vi "EV Rotator Shutdown Editor.vi"(6 "Channel":i32=1, 8 "Calibration in":string, 9 "Hardware in":string, 10 "Setup in":string, 11 "Editor seq info":T1 {"Steps config"."Loop Info"."unit scale" items=["Log", "Lin"]; "Steps config"."Loop Info"."unit dB ref" format="%#_6p"}) -> (1 "Step name out":string="Calibration Default", 2 "Setup out":string, 3 "Sequence channels & curves out":string[](array[string]))   [LabVIEW 2018]
uses:
  custom and Sc run Seq Sub VIs (x64).llb/editor seq info.ctl
  custom and Sc run Seq Sub VIs (x64).llb/Steps config.ctl
  C:/SoundCheck 19/System/Custom VIs/EV.Rotator.RotatorControl.dll
  EV.Rotator.RotatorControl.dll
panel:
  out "Rotator Control.dll version":string
  in  "Save as":bool
  in  "save":bool
  in  "revert":bool
  in  "continue loop?":bool
  in  "cancel":bool
  in  "load":bool
  # "This VI runs the following shutdown routine:\n  - disables absolute movement mode\n  - disables drives\n  - enables Ab mode\n  - disables Ab mode"
  # "Reminder:  You must edit this custom step from\nwithin a sequence for it to remember your settings."
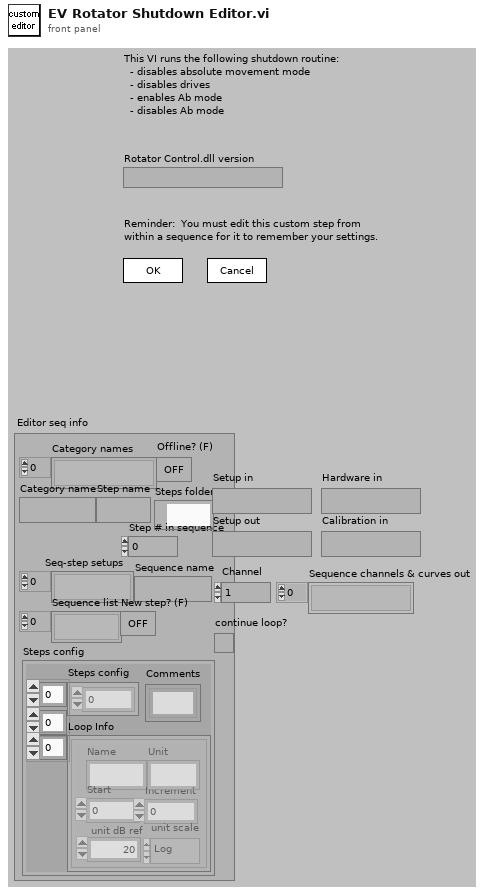
[diagram p1: front panel]
types:
  T1 = typedef "editor seq info.ctl" = cluster{"Category names":string[], "Category name":string, "Step name":string, "Step # in sequence":i32, "Seq-step setups":string[], "Sequence name":string, "Sequence list":string[], "New step? (F)":bool, "Steps config":T2, "Offline? (F)":bool, "Steps folder":path}
  T2 = typedef "Steps config.ctl" = cluster{"Steps config":i32[][], "Loop Info":cluster{"Name":string, "Start":dbl, "Increment":dbl, "Unit":string, "unit dB ref":dbl, "unit scale":u16}[], "Comments":string[]}
  T3 = cluster{"load":bool, "revert":bool, bool, "cancel":bool, "Save as":bool, bool, bool}
  T4 = cluster{"load":bool, "revert":bool, "save":bool, "cancel":bool, "Save as":bool, "close panel":bool, "apply":bool}
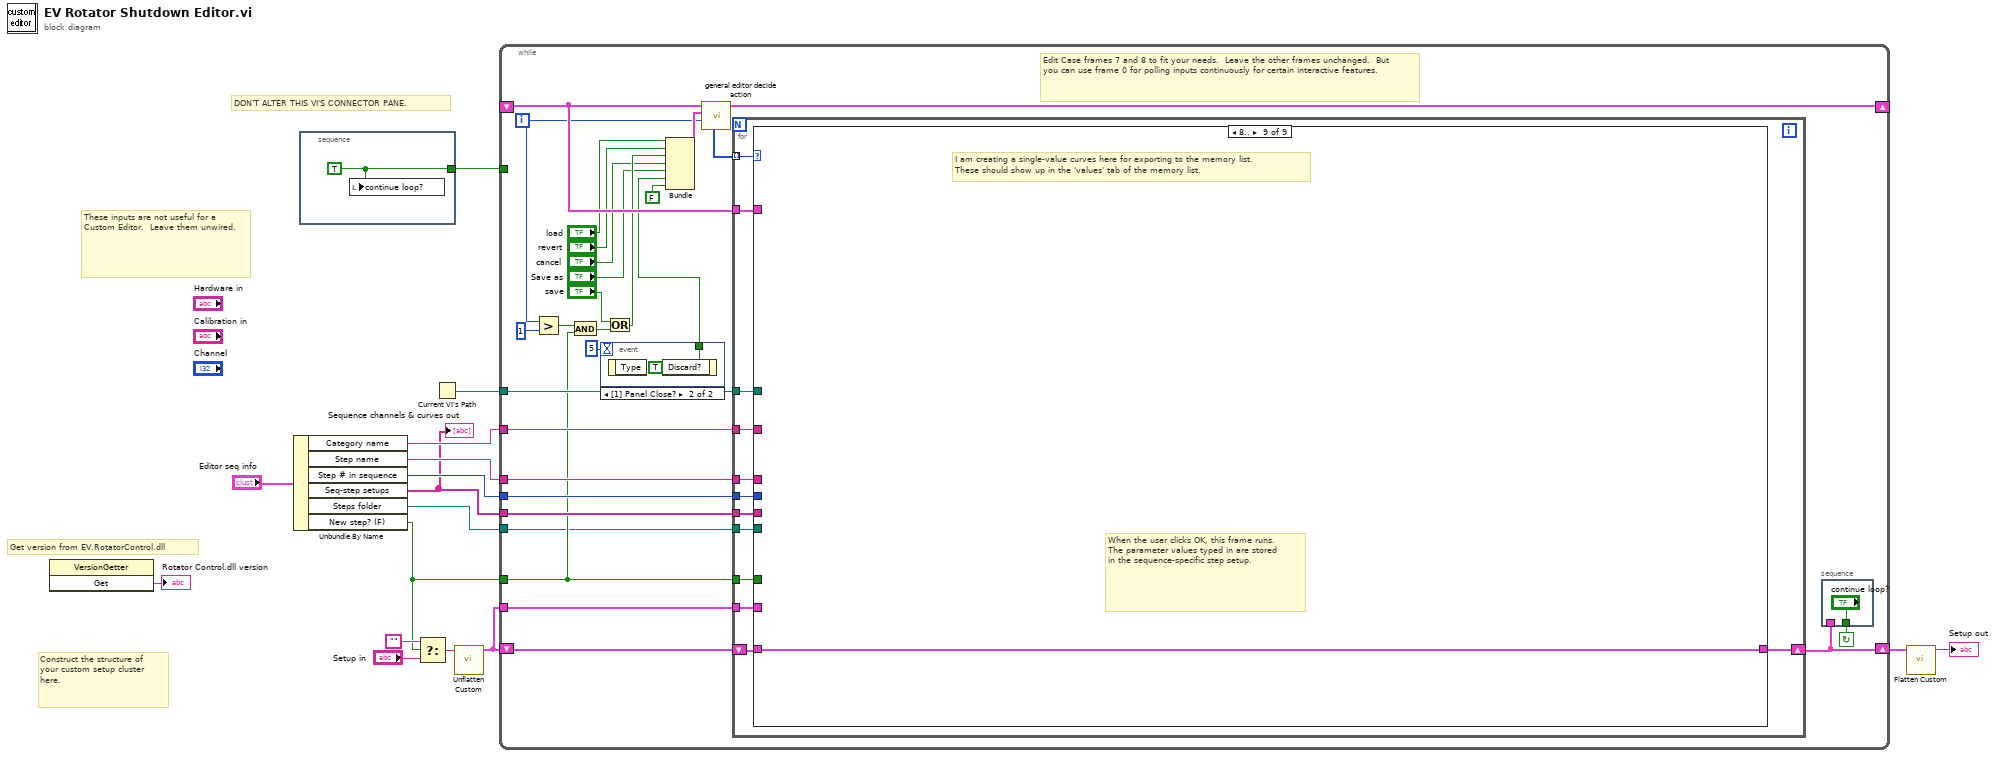
[diagram p0: block diagram]
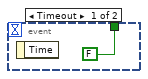
[diagram p2: hidden frame]
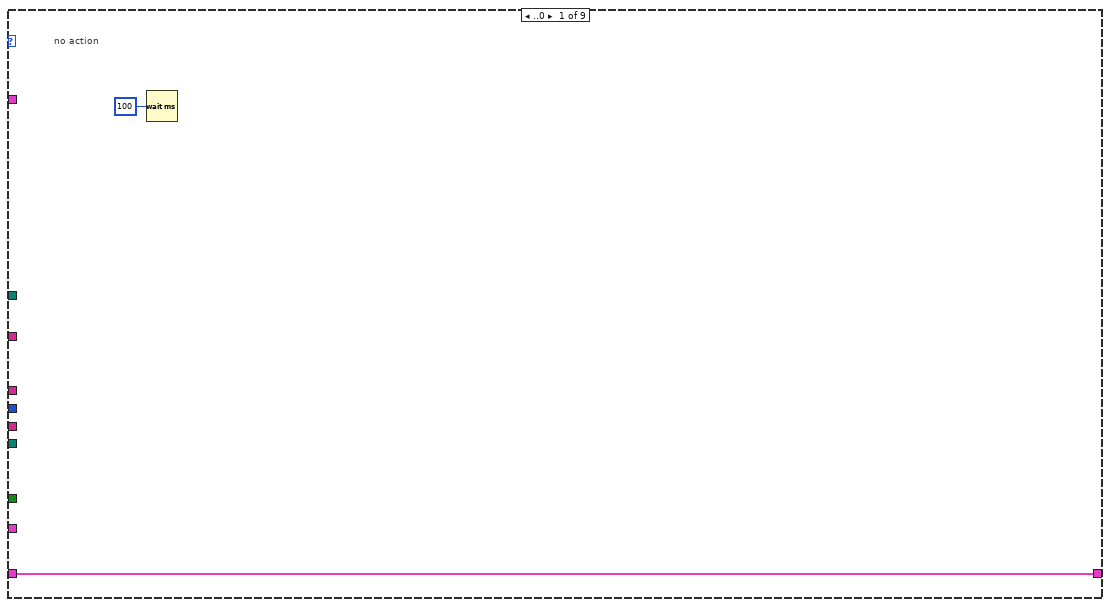
[diagram p3: hidden frame]
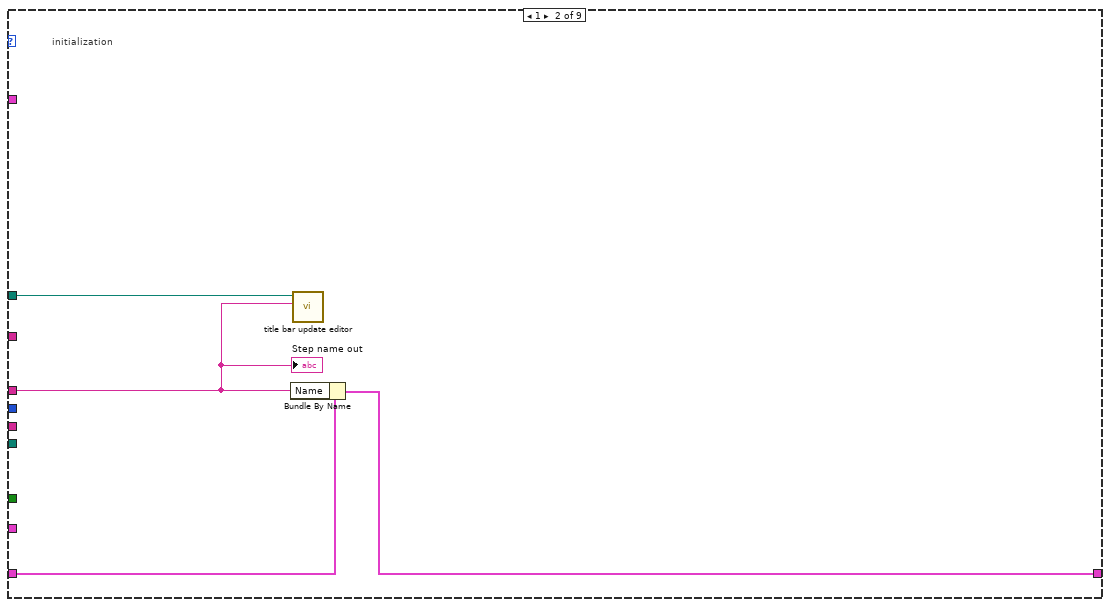
[diagram p4: hidden frame]
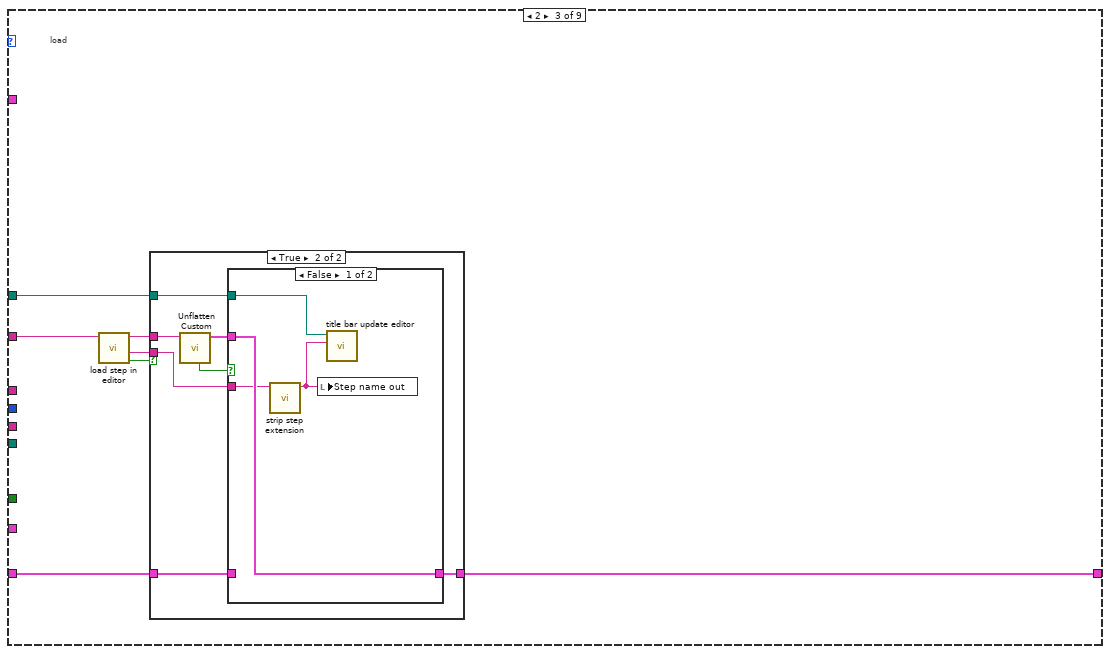
[diagram p5: hidden frame]
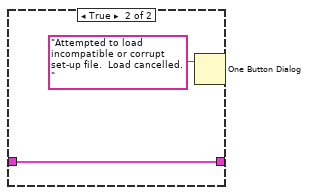
[diagram p7: hidden frame]
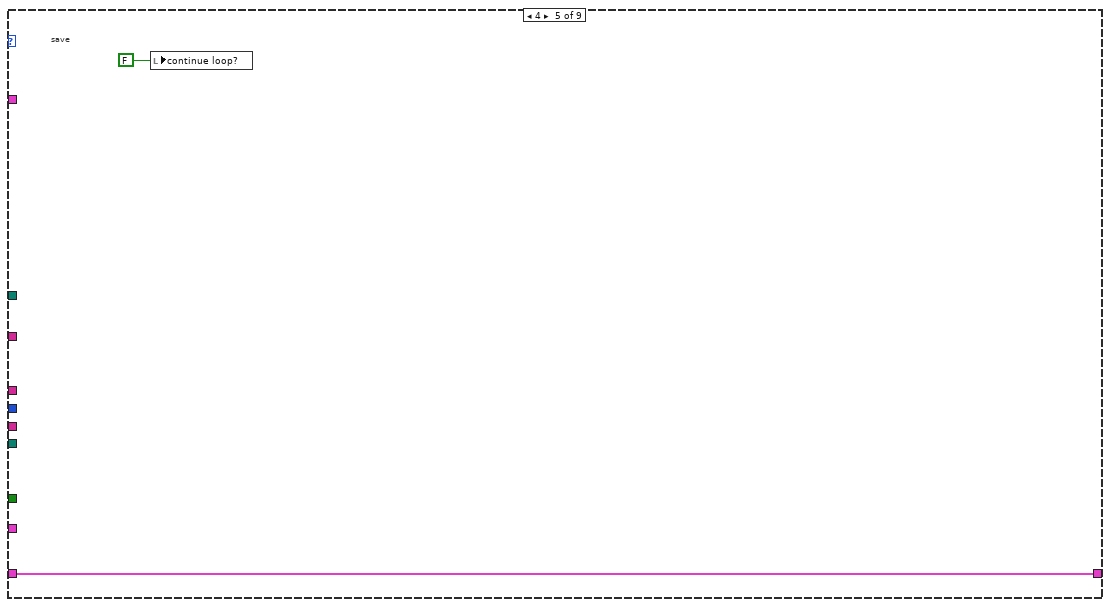
[diagram p9: hidden frame]
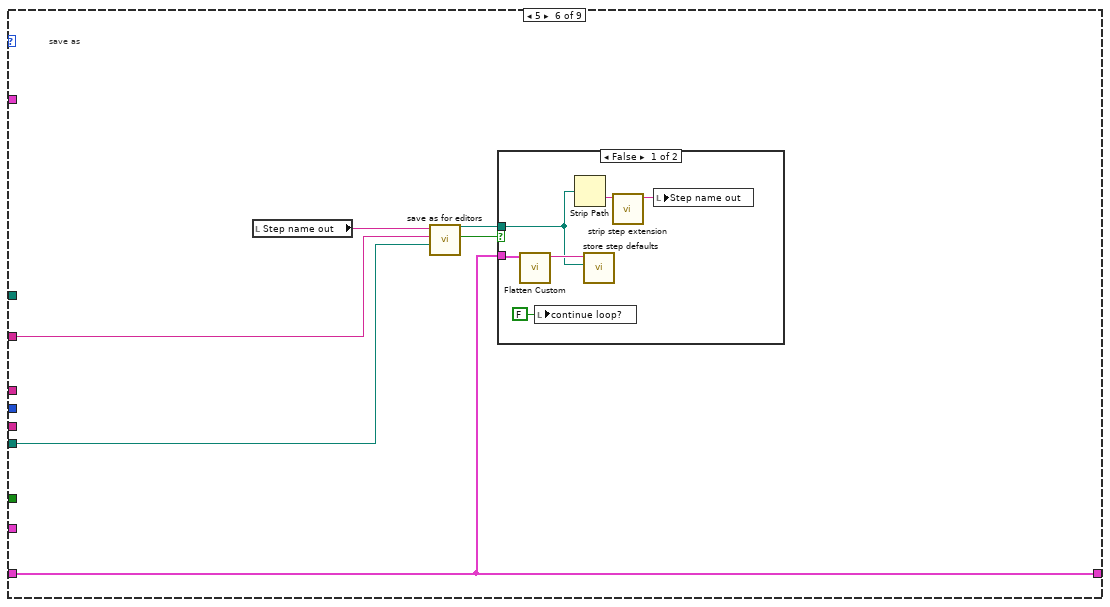
[diagram p10: hidden frame]
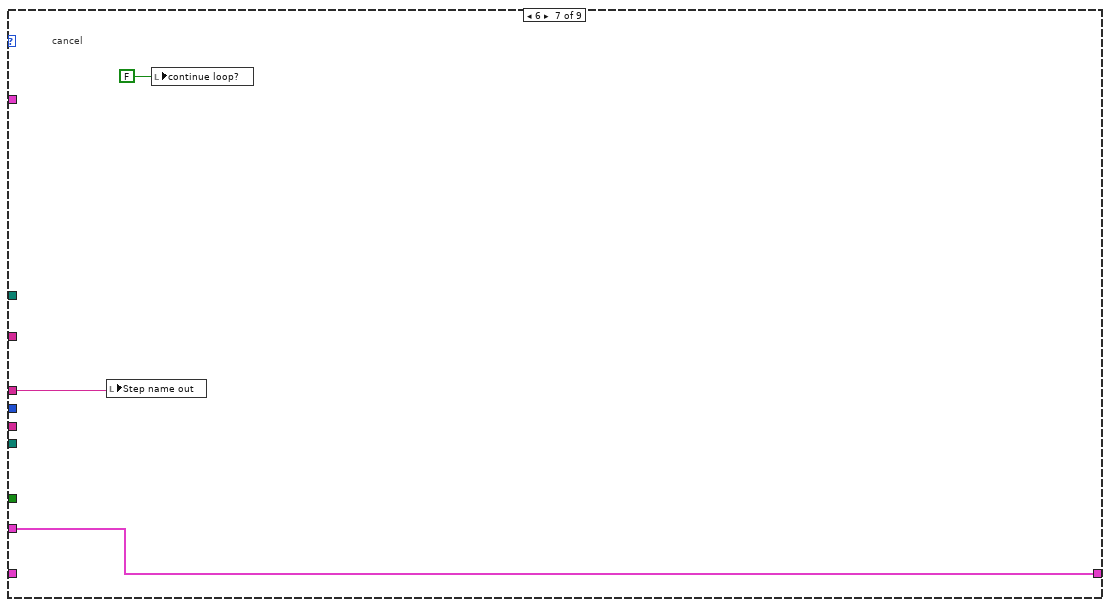
[diagram p12: hidden frame]
diagram:
  # "Get version from EV.RotatorControl.dll"
  # "Construct the structure of your custom setup cluster here."
  # "These inputs are not useful for a Custom Editor.  Leave them unwired."
  # "DON'T ALTER THIS VI'S CONNECTOR PANE."
  n1 = invoke class="VersionGetter" method="Get"() -> ("Get"=→"Rotator Control.dll version":string)  [unwired: 3 in, 2 out]
  n2 = Unbundle By Name("Editor seq info") -> ("Category name"=w10:string, "Step name"=w9:string, "Step # in sequence"=w8:i32, "Seq-step setups"=w6:string[], "Steps folder"=w7:path, "New step? (F)"=w3:bool)
  "Sequence channels & curves out" <- w6
  n3 = stacked-sequence {
    tunnel: [w17] -> w11
    frame #0 {
      w17 = TRUE ("continue loop?")
      n4 = local write "continue loop?"(w17) -> ()
    }
  }
  n5 = Select(t="", s=w3, f="Setup in") -> (s? t:f=w13:string)
  n6 = Current VI's Path() -> (path=w12:path)
  n7 = call "Unflatten Custom.vi"("Unflatten Custom"=w13) -> ("Custom"=w2:cluster{"Name":string})  [unwired: 10 out]
  n8 = while {
    tunnel: w12 -> [w34]
    shift-left: w2 -> [w36]
    shift-right: [w27] -> w4
    tunnel: w2 -> [w38]
    tunnel: w3 -> [w30]
    tunnel: w6 -> [w40]
    tunnel: w8 -> [w41]
    tunnel: w9 -> [w42]
    tunnel: w10 -> [w43]
    shift-left: _ -> [w37]
    shift-right: [w45] -> _
    tunnel: w7 -> [w24]
    tunnel: w11 -> [_]
    i -> [w33]
    stop <- w39 continue-if-true
    # "Edit Case frames 7 and 8 to fit your needs.  Leave the other frames unchanged.  But you can use frame 0 for polling inputs continuously for certain interactive features."
    n9 = Greater?(x=w33, y=1) -> (0:w31:bool)
    n10 = And(x=w31, y=w30) -> (x .and. y?=w29:bool)
    n11 = event shown="[1] Panel Close?" {
      selector: _ -> [_ _]
      dyn-events: _ -> [_ _]
      timeout: 5 -> [_ _]
      tunnel: [FALSE w47] -> w26
      event Timeout {
        n12 = event-data() -> ()  [unwired: 2 out]
      }
      event Panel Close? {
        w47 = TRUE
        n13 = event-data() -> ()  [unwired: 2 out]
        n14 = event-data("Discard?"=w47) -> ()  [unwired: 1 in, 1 out]
      }
    }
    n15 = Or(x="save", y=w29) -> (x .or. y?=w28:bool)
    n16 = Bundle("load"="load", "revert"="revert", w28, "cancel"="cancel", "Save as"="Save as", w26, FALSE) -> (w35:T3)  [unwired: 1 out]
    n17 = call "general editor decide action.vi"("Iteration"=w33, "Polled cluster"=w35, "Old cluster"=w37) -> ("actions array"=w44:i32[], "New cluster"=w45:T4)  [unwired: 1 in, 6 out]
    n18 = for {
      tunnel: w37 -> [w60]
      tunnel: w38 -> [w59]
      tunnel: w30 -> [w58]
      tunnel: w40 -> [w57]
      tunnel: w41 -> [w56]
      tunnel: w42 -> [w55]
      tunnel: w43 -> [w54]
      tunnel: w44 -> [w53] mode=indexing
      shift-right: [w51] -> w27
      shift-left: w36 -> [w52]
      tunnel: w34 -> [w50]
      tunnel: w24 -> [w49]
      n19 = case shown="8.." w53 {
        tunnel: w54 -> [_ _ w69 _ _ w93 _ _ _]
        tunnel: w55 -> [_ w63 _ _ _ _ w103 _ _]
        tunnel: w56 -> [_ _ _ _ _ _ _ _ _]
        tunnel: w57 -> [_ _ _ _ _ _ _ _ _]
        tunnel: w58 -> [_ _ _ _ _ _ _ _ _]
        tunnel: w59 -> [_ _ _ w88 _ _ w104 _ _]
        tunnel: [w61 w66 w73 w88 w89 w96 w104 w106 w107] -> w51
        tunnel: w52 -> [w61 w65 w72 _ w89 w96 _ w106 w107]
        tunnel: w60 -> [_ _ _ _ _ _ _ _ _]
        tunnel: w50 -> [_ w64 w67 _ _ _ _ _ _]
        tunnel: w49 -> [_ _ _ _ _ w91 _ _ _]
        frame ..0 {
          # "no action"
          n20 = Wait (ms)(milliseconds to wait=u32 100) -> ()  [unwired: 1 out]
        }
        frame 1 {
          # "initialization"
          n21 = Bundle By Name(cluster=w65, "Name"=w63) -> (w66:cluster{"Name":string})
          n22 = call "title bar update editor.vi"("Step name"=w63, "Editor VI path"=w64) -> ()  [unwired: 10 out]
          "Step name out" <- w63
        }
        frame 2 {
          # "load"
          n23 = call "load step in editor.vi"("Category name"=w69) -> ("Not canceled?"=w70:bool, "New step name (with ext.)"=w68:string, "Flat step set-up"=w71:string)  [unwired: 1 in, 7 out]
          n24 = case shown="True" w70 {
            tunnel: w71 -> [_ w81]
            tunnel: [w74 w79] -> w73
            tunnel: w72 -> [w74 w78]
            tunnel: w68 -> [_ w76]
            tunnel: w67 -> [_ w75]
            frame False {
            }
            frame True {
              n25 = call "Unflatten Custom.vi"("Unflatten Custom"=w81) -> ("Custom"=w77:cluster{"Name":string}, "Error?"=w80:bool)  [unwired: 9 out]
              n26 = case shown="False" w80 {
                tunnel: [w85 w87] -> w79
                tunnel: w78 -> [_ w87]
                tunnel: w77 -> [w85 _]
                tunnel: w76 -> [w84 _]
                tunnel: w75 -> [w83 _]
                frame False {
                  n27 = call "strip step extension.vi"("Step name w/ extension"=w84) -> ("Step name (base)"=w82:string)  [unwired: 1 in, 9 out]
                  n28 = local write "Step name out"(w82) -> ()
                  n29 = call "title bar update editor.vi"("Step name"=w82, "Editor VI path"=w83) -> ()  [unwired: 10 out]
                }
                frame True {
                  n30 = One Button Dialog(message="Attempted to load incompatible or corrupt set-up file.  Load cancelled.") -> ()  [unwired: 2 out]
                }
              }
            }
          }
        }
        frame 3 {
          # "revert"
        }
        frame 4 {
          # "save"
          n31 = local write "continue loop?"(FALSE ("continue loop?")) -> ()
        }
        frame 5 {
          # "save as"
          n32 = local read "Step name out"() -> (w92:string)
          n33 = call "save as for editors.vi"("Steps Folder (gbl if empty)"=w91, "Category name"=w93, "Step name"=w92) -> ("Canceled"=w94:bool, "File path chosen"=w95:path)  [unwired: 3 in, 4 out]
          n34 = case shown="False" w94 {
            tunnel: w95 -> [w98 _]
            tunnel: w96 -> [w101 _]
            frame False {
              n35 = call "Flatten Custom.vi"("Custom"=w101) -> ("Custom flattened"=w102:string)  [unwired: 10 out]
              n36 = local write "continue loop?"(FALSE ("continue loop?")) -> ()
              n37 = Strip Path(path=w98) -> (name=w99:string)  [unwired: 1 out]
              n38 = call "store step defaults.vi"("Set-up file"=w98, "Flat step set-up"=w102) -> ()  [unwired: 4 in, 6 out]
              n39 = call "strip step extension.vi"("Step name w/ extension"=w99) -> ("Step name (base)"=w97:string)  [unwired: 1 in, 9 out]
              n40 = local write "Step name out"(w97) -> ()
            }
            frame True {
            }
          }
        }
        frame 6 {
          # "cancel"
          n41 = local write "Step name out"(w103) -> ()
          n42 = local write "continue loop?"(FALSE ("continue loop?")) -> ()
        }
        frame 7 {
          # "When this editor VI runs, it first writes the parameter values to the front panel.  The values are saved in the sequence-specific step setup for the current sequence.  If an error occurs extracting the values, write default values as shown."
          # "update set-up data"
        }
        frame 8.. {
          # "I am creating a single-value curves here for exporting to the memory list.\nThese should show up in the 'values' tab of the memory list."
          # "When the user clicks OK, this frame runs.  The parameter values typed in are stored in the sequence-specific step setup."
        }
      }
    }
    n43 = stacked-sequence {
      tunnel: ["continue loop?"] -> w39
      tunnel: w27 -> [_]
      frame #0 {
      }
    }
  }
  n44 = call "Flatten Custom.vi"("Custom"=w4) -> ("Custom flattened"=→"Setup out":string)  [unwired: 10 out]
